vi "setCellType.vi"(0 "MS-Excel in":refnum<class "MS-Excel.lvclass">, 5 "Cell Type":i32(ring)=1 items=["Numeric"=0, "String"=1, "Formula"=2, "Blank"=3, "Boolean"=4, "Error"=5, "Unknown"=-1], 7 "Start":cluster{"Row":i32, "Column":i32}, 9 "End":cluster{"Row":i32, "Column":i32}, 11 "error in (no error)":errorcluster) -> (4 "MS-Excel out":refnum<class "MS-Excel.lvclass">, 15 "error out":errorcluster)   [LabVIEW 2017, in "LabVIEW NPOI.lvlib" / "MS-Excel.lvclass"]
uses:
  MS-Excel.lvclass
  MS-Excel.lvclass/MS-Excel.ctl
  C:/Users/Neo/Desktop/Dev_Tools_BR/LabVIEW_NPOI/lib/NPOI 2.1.1/NPOI.dll
  lib/NPOI 2.1.1/NPOI.dll
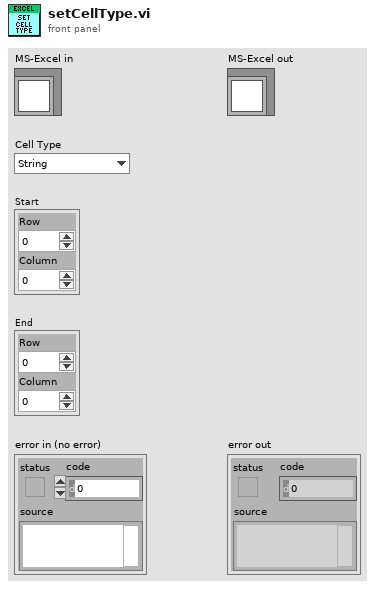
[diagram p1: front panel]
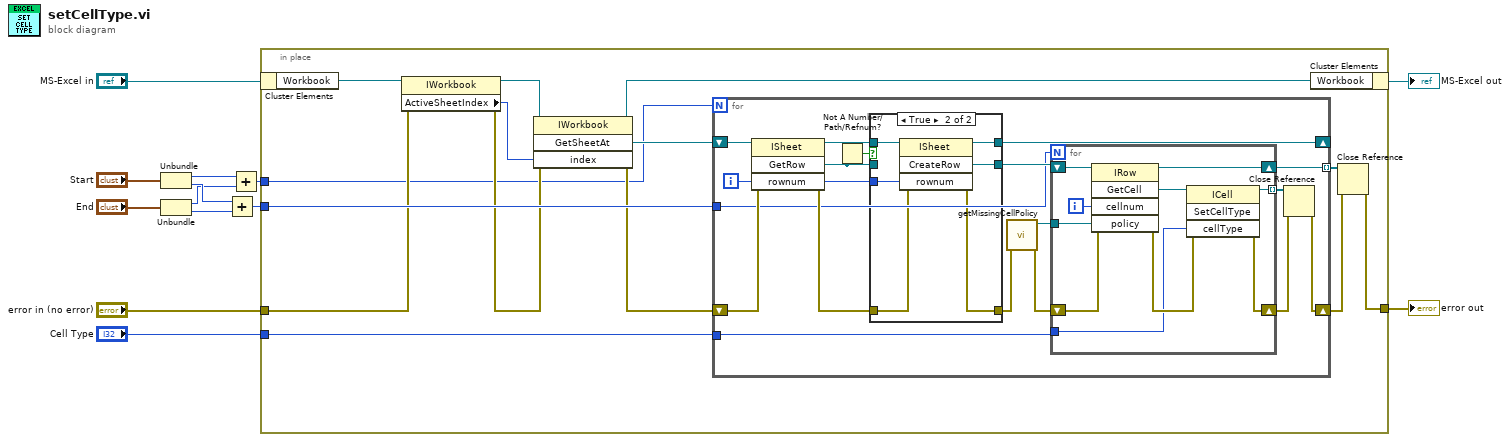
[diagram p0: block diagram]
diagram:
  n1 = Unbundle("Start") -> ("Row"=w8:i32, "Column"=w10:i32)
  n2 = Unbundle("End") -> ("Row"=w9:i32, "Column"=w11:i32)
  n3 = Add(x=w10, y=w11) -> (x+y=w6:i32)
  n4 = Add(x=w8, y=w9) -> (x+y=w7:i32)
  n5 = in-place {
    in-place-border: "error in (no error)" -> [w17]
    in-place-border: [w23] -> w1
    in-place-border: w7 -> [w15]
    in-place-border: w6 -> [w26]
    in-place-border: "Cell Type" -> [w14]
    n6 = in-place-cluster #1("MS-Excel in") -> ("Workbook"=w27:refnum<k24>)
    n7 = property class="IWorkbook"(reference=w27, error in=w17) -> (reference out=w19:refnum<k24>, error out=w16:errorcluster, "ActiveSheetIndex"=w18:i32)
    n8 = invoke class="IWorkbook" method="GetSheetAt"(reference=w19, error in=w16, "index"=w18) -> (reference out=w21:refnum<k24>, error out=w20:errorcluster, "GetSheetAt"=w22:refnum<k24>)  [unwired: 1 in, 1 out]
    n9 = for {
      N: w15 -> [_]
      shift-right: [w41] -> _
      shift-left: w22 -> [w45]
      shift-right: [w35] -> w24
      shift-left: w20 -> [w39]
      tunnel: w26 -> [w30]
      tunnel: [w34] -> w25 mode=indexing
      tunnel: w14 -> [w28]
      i -> [w29]
      n10 = invoke class="ISheet" method="GetRow"(reference=w45, error in=w39, "rownum"=w29) -> (reference out=w42:refnum<k24>, error out=w40:errorcluster, "GetRow"=w43:refnum<k24>)  [unwired: 1 in, 1 out]
      n11 = Not A Number/Path/Refnum?(number/path/refnum=w43) -> (NaN/Path/Refnum?=w44:bool)
      n12 = case shown="True" w44 {
        tunnel: w43 -> [w57 _]
        tunnel: w42 -> [w56 w64]
        tunnel: w29 -> [_ w63]
        tunnel: w40 -> [w58 w59]
        tunnel: [w58 w61] -> w32
        tunnel: [w57 w62] -> w38
        tunnel: [w56 w60] -> w41
        frame False {
        }
        frame True {
          n13 = invoke class="ISheet" method="CreateRow"(reference=w64, error in=w59, "rownum"=w63) -> (reference out=w60:refnum<k24>, error out=w61:errorcluster, "CreateRow"=w62:refnum<k24>)  [unwired: 1 in, 1 out]
        }
      }
      n14 = call "getMissingCellPolicy.vi"("error in (no error)"=w32) -> ("error out"=w31:errorcluster, "CREATE_NULL_AS_BLANK"=w33:refnum<k24>)  [unwired: 9 in]
      n15 = for {
        N: w30 -> [_]
        shift-right: [w54] -> w34
        shift-left: w38 -> [w55]
        shift-right: [w52] -> w36
        shift-left: w31 -> [w53]
        tunnel: [w51] -> w37 mode=indexing
        tunnel: w33 -> [w50]
        tunnel: w28 -> [w46]
        i -> [w48]
        n16 = invoke class="IRow" method="GetCell"(reference=w55, error in=w53, "cellnum"=w48, "policy"=w50) -> (reference out=w54:refnum<k24>, error out=w47:errorcluster, "GetCell"=w49:refnum<k24>)  [unwired: 1 in, 2 out]
        n17 = invoke class="ICell" method="SetCellType"(reference=w49, error in=w47, "cellType"=w46) -> (reference out=w51:refnum<k24>, error out=w52:errorcluster)  [unwired: 1 in, 2 out]
      }
      n18 = Close Reference(reference=w37, error in (no error)=w36) -> (error out=w35:errorcluster)
    }
    n19 = in-place-cluster #1("Workbook"=w21) -> (→"MS-Excel out":refnum<class "MS-Excel.lvclass">)
    n20 = Close Reference(reference=w25, error in (no error)=w24) -> (error out=w23:errorcluster)
  }
  "error out" <- w1
